vi "Atuador Y.vi"(8 "error in (no error)":errorcluster, 10 "Parameters In":variant, 11 "Subpanel Queue In":refnum<queue>) -> (0 "error out":errorcluster, 2 "Parameters Out":variant)   [LabVIEW 2018]
doc: "Configuration control for the 'Hold' step."
panel:
  in  "Enum":T1(ring)
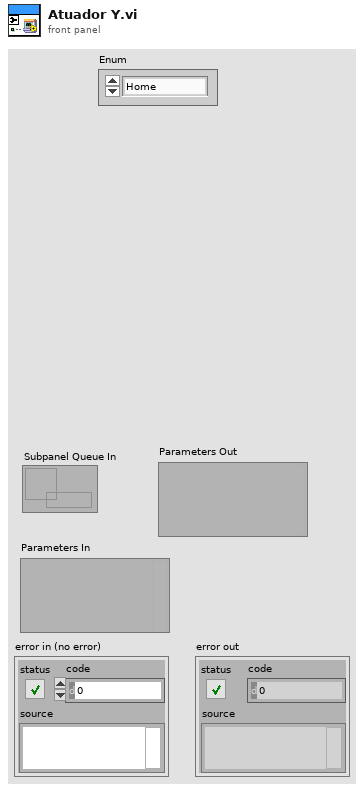
[diagram p1: front panel]
types:
  T1 = enum16{"Home", "Carregamento", "Inspeção 1", "Inspeção 2"}
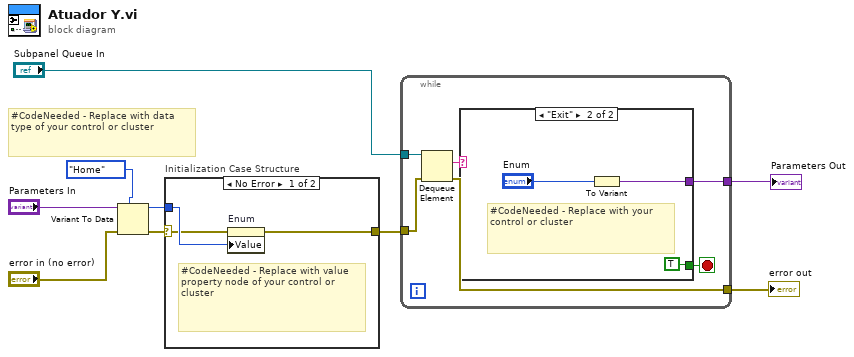
[diagram p0: block diagram]
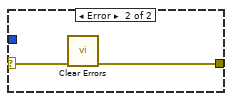
[diagram p2: hidden frame]
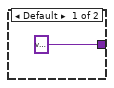
[diagram p3: hidden frame]
diagram:
  # "#CodeNeeded - Replace with data type of your control or cluster"
  n1 = Variant To Data(error in="error in (no error)", type=T1."Home" ("Enum"), Variant="Parameters In") -> (data=w7:T1, error out=w5:errorcluster)
  n2 = case "Initialization Case Structure" shown="No Error" w5 {
    selector: w5 -> [w11 w14]
    tunnel: w7 -> [w12 _]
    tunnel: [w10 w13] -> w6
    frame No Error {
      # "#CodeNeeded - Replace with value property node of your control or cluster"
      n3 = property on="Enum" class="Enum (strict)"(error in=w11, "Value"=w12) -> (error out=w10:errorcluster)  [unwired: 1 in, 1 out]
    }
    frame Error {
      n4 = call <vilib>:"Clear Errors.vi"("error in (no error)"=w14) -> ("error out"=w13:errorcluster)  [unwired: 5 in, 1 out]
    }
  }
  n5 = while {
    tunnel: "Subpanel Queue In" -> [w20]
    tunnel: w6 -> [w19]
    tunnel: [w17] -> w4
    tunnel: [w15] -> w2
    stop <- w16 stop-if-true
    n6 = Dequeue Element(queue=w20, error in (no error)=w19) -> (element=w18:string, error out=w15:errorcluster)  [unwired: 1 in, 2 out]
    n7 = case shown="\"Exit\"" w18 {
      tunnel: [variant ("Variant") w24] -> w17
      tunnel: [_ TRUE] -> w16
      frame Default {
      }
      frame "Exit" {
        # "#CodeNeeded - Replace with your control or cluster"
        n8 = To Variant(anything="Enum") -> (Variant=w24:variant)
      }
    }
  }
  "Parameters Out" <- w4
  "error out" <- w2
